vi "PIXY VI.vi"() -> (14 "BLOCK":dbl, 15 "SIG":dbl, 16 "X":dbl, 17 "WIDTH":dbl, 18 "Y":dbl, 19 "HEIGHT":dbl)   [LabVIEW 2017]
uses:
  <vilib>/Rock Robotics/Network Tables/NT Read String.vi
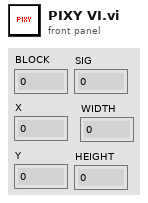
[diagram p1: front panel]
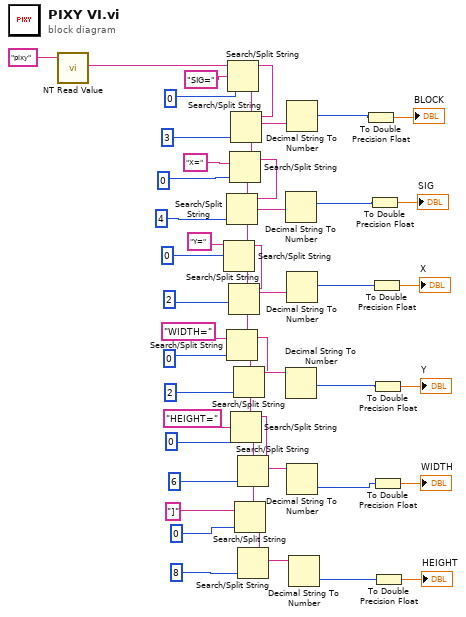
[diagram p0: block diagram]
diagram:
  n1 = call-poly <vilib>:"NT Read Value.vi"("Name"="pixy") -> ("String"=w48:string)  [unwired: 9 in, 1 out]
  n2 = Search/Split String(string=w48, search string/char (-)="SIG=", offset (0)=0) -> (substring before match=w13:string, match + rest of string=w45:string)  [unwired: 1 out]
  n3 = Search/Split String(string=w45, search string/char (-)="X=", offset (0)=0) -> (substring before match=w16:string, match + rest of string=w42:string)  [unwired: 1 out]
  n4 = Search/Split String(string=w42, search string/char (-)="Y=", offset (0)=0) -> (substring before match=w20:string, match + rest of string=w39:string)  [unwired: 1 out]
  n5 = Search/Split String(string=w16, offset (0)=4) -> (match + rest of string=w17:string)  [unwired: 1 in, 2 out]
  n6 = Search/Split String(string=w39, search string/char (-)="WIDTH=", offset (0)=0) -> (substring before match=w22:string, match + rest of string=w36:string)  [unwired: 1 out]
  n7 = Search/Split String(string=w20, offset (0)=2) -> (match + rest of string=w21:string)  [unwired: 1 in, 2 out]
  n8 = Search/Split String(string=w13, offset (0)=3) -> (match + rest of string=w14:string)  [unwired: 1 in, 2 out]
  n9 = Search/Split String(string=w36, search string/char (-)="HEIGHT=", offset (0)=0) -> (substring before match=w26:string, match + rest of string=w33:string)  [unwired: 1 out]
  n10 = Search/Split String(string=w22, offset (0)=2) -> (match + rest of string=w23:string)  [unwired: 1 in, 2 out]
  n11 = Search/Split String(string=w33, search string/char (-)="]", offset (0)=0) -> (substring before match=w29:string)  [unwired: 2 out]
  n12 = Search/Split String(string=w26, offset (0)=6) -> (match + rest of string=w25:string)  [unwired: 1 in, 2 out]
  n13 = Search/Split String(string=w29, offset (0)=8) -> (match + rest of string=w28:string)  [unwired: 1 in, 2 out]
  n14 = Decimal String To Number(string=w17) -> (number=w7:i32)  [unwired: 2 in, 1 out]
  n15 = Decimal String To Number(string=w23) -> (number=w9:i32)  [unwired: 2 in, 1 out]
  n16 = Decimal String To Number(string=w14) -> (number=w12:i32)  [unwired: 2 in, 1 out]
  n17 = Decimal String To Number(string=w21) -> (number=w8:i32)  [unwired: 2 in, 1 out]
  n18 = Decimal String To Number(string=w25) -> (number=w11:i32)  [unwired: 2 in, 1 out]
  n19 = Decimal String To Number(string=w28) -> (number=w10:i32)  [unwired: 2 in, 1 out]
  n20 = To Double Precision Float(number=w12) -> (double precision float=→"BLOCK":dbl)
  n21 = To Double Precision Float(number=w7) -> (double precision float=→"SIG":dbl)
  n22 = To Double Precision Float(number=w8) -> (double precision float=→"X":dbl)
  n23 = To Double Precision Float(number=w9) -> (double precision float=→"Y":dbl)
  n24 = To Double Precision Float(number=w11) -> (double precision float=→"WIDTH":dbl)
  n25 = To Double Precision Float(number=w10) -> (double precision float=→"HEIGHT":dbl)
